vi "Merge Tokens of Ini Files.vi"(8 "error in (no error)":errorcluster, 11 "Path":path) -> (0 "error out":errorcluster)   [LabVIEW 2020]
doc: "Use this template to build a VI to use as a subVI."
uses:
  <vilib>/Utility/config.llb/Read Key (String).vi
  <vilib>/Utility/config.llb/NI_LVConfig.lvlib
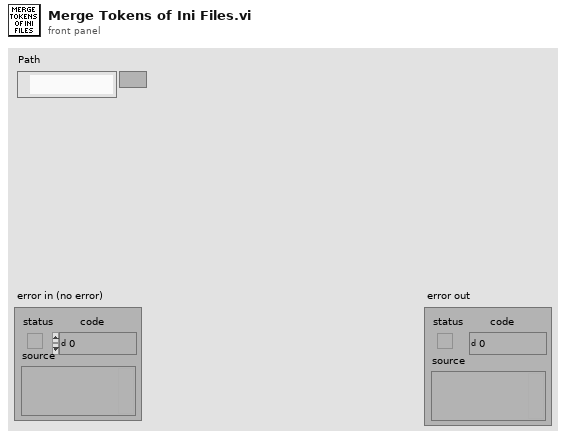
[diagram p1: front panel]
types:
  T1 = typedef "NI_LVConfig.lvlib/Config Data RefNum.ctl" = refnum<k1>
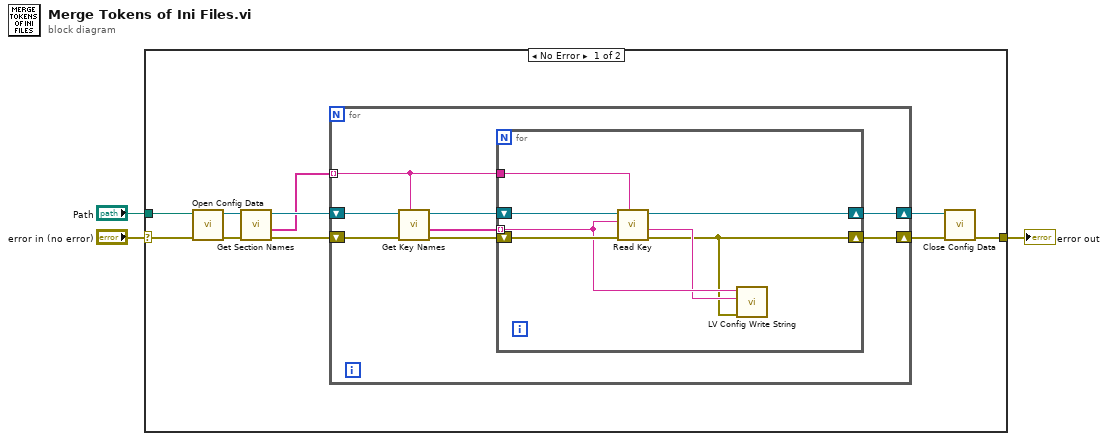
[diagram p0: block diagram]
diagram:
  n1 = case shown="No Error" "error in (no error)" {
    selector: "error in (no error)" -> [w9 w29]
    tunnel: [w4 w29] -> w2
    tunnel: "Path" -> [w10 _]
    frame No Error {
      n2 = call <vilib>:"Open Config Data.vi"("error in (no error)"=w9, "configuration file path"=w10) -> ("error out"=w7:errorcluster, "refnum"=w13:T1)  [unwired: 7 in, 1 out]
      n3 = call <vilib>:"Get Section Names.vi"("error in (no error)"=w7, "refnum"=w13) -> ("error out"=w6:errorcluster, "section names"=w5:string[], "refnum out"=w8:T1)  [unwired: 7 in]
      n4 = for {
        shift-right: [w20] -> w11
        shift-left: w8 -> [w21]
        shift-right: [w19] -> w12
        shift-left: w6 -> [w17]
        tunnel: w5 -> [w15] mode=indexing
        n5 = call <vilib>:"Get Key Names.vi"("section"=w15, "error in (no error)"=w17, "refnum"=w21) -> ("error out"=w16:errorcluster, "key names"=w14:string[], "refnum out"=w18:T1)  [unwired: 5 in, 1 out]
        n6 = for {
          tunnel: w15 -> [w25]
          tunnel: w14 -> [w24] mode=indexing
          shift-right: [w28] -> w20
          shift-left: w18 -> [w27]
          shift-right: [w22] -> w19
          shift-left: w16 -> [w26]
          n7 = call-poly <vilib>:"Read Key.vi"("section"=w25, "error in (no error)"=w26, "key"=w24, "refnum"=w27) -> ("error out"=w22:errorcluster, "value"=w23:string, "refnum out"=w28:T1)  [unwired: 4 in, 1 out]
          n8 = call <resource>:"LV Config Write String.vi"("error in (no error)"=w22, "value"=w23, "key"=w24) -> ()  [unwired: 4 in, 1 out]
        }
      }
      n9 = call <vilib>:"Close Config Data.vi"("error in (no error)"=w12, "refnum"=w11) -> ("error out"=w4:errorcluster)  [unwired: 8 in, 1 out]
    }
    frame Error {
    }
  }
  "error out" <- w2
